vi "WCET Write To File.vi"(10 "Path":path=path "C:/Users/ReCog/Desktop/WCET.txt", 11 "Statistical Metrics":dbl[](array[numeric])) -> (0 "Error out":errorcluster)   [LabVIEW 2020]
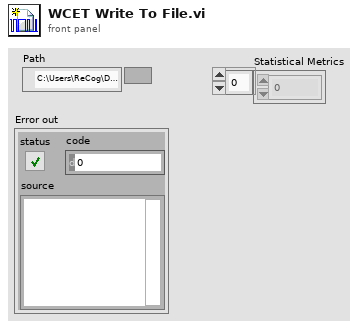
[diagram p1: front panel]
types:
  T1 = enum16{"open", "replace", "create", "open or create", "replace or create", "replace or create with confirmation"}
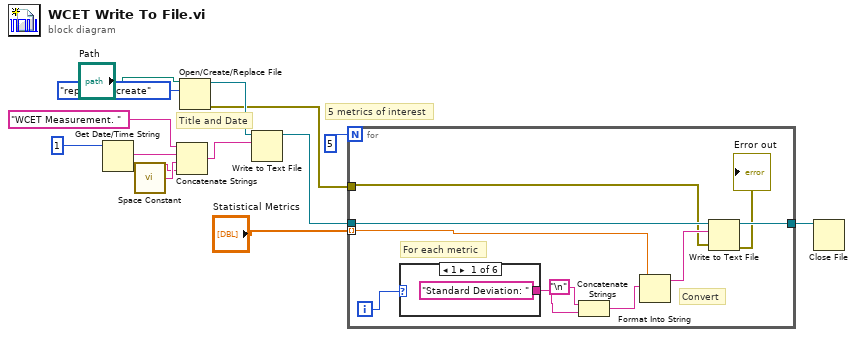
[diagram p0: block diagram]
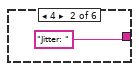
[diagram p2: hidden frame]
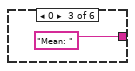
[diagram p3: hidden frame]
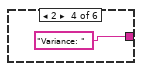
[diagram p4: hidden frame]
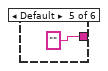
[diagram p5: hidden frame]
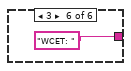
[diagram p6: hidden frame]
diagram:
  # "5 metrics of interest"
  # "Title and Date"
  n1 = Get Date/Time String(date format (0)=1) -> (date string=w9:string, time string=w13:string)  [unwired: 2 in]
  n2 = call <vilib>:"Space Constant.vi"() -> ("String"=w14:string)
  n3 = Concatenate Strings("WCET Measurement. ", w9, w14, w13) -> (w11:string)
  n4 = Open/Create/Replace File(file path (use dialog)="Path", operation (0:open)=T1."replace or create") -> (refnum out=w7:refnum<file>, error out=w4:errorcluster)  [unwired: 4 in, 1 out]
  n5 = Write to Text File(file (use dialog)=w7, text=w11) -> (refnum out=w12:refnum<file>)  [unwired: 2 in, 2 out]
  n6 = for {
    N: 5 -> [_]
    tunnel: w12 -> [w24]
    tunnel: [w22] -> w5
    tunnel: w4 -> [w21]
    tunnel: "Statistical Metrics" -> [w20] mode=indexing
    i -> [w18]
    # "Convert"
    # "For each metric"
    n7 = case shown="1" w18 {
      tunnel: ["Standard Deviation: " "Jitter: " "Mean: " "Variance: " "" "WCET: "] -> w15
      frame 1 {
      }
      frame 4 {
      }
      frame 0 {
      }
      frame 2 {
      }
      frame Default {
      }
      frame 3 {
      }
    }
    n8 = Concatenate Strings("\n", w15) -> (w17:string)
    n9 = Format Into String(initial string=w17, w20) -> (resulting string=w23:string)  [unwired: 2 in, 1 out]
    n10 = Write to Text File(file (use dialog)=w24, text=w23, error in=w21) -> (refnum out=w22:refnum<file>, error out=→"Error out":errorcluster)  [unwired: 1 in, 1 out]
  }
  n11 = Close File(refnum=w5) -> ()  [unwired: 1 in, 2 out]
